vi "Read Compatible Hardware Table.vi"(8 "error in (no error)":errorcluster, 11 "Mag Lab Measure Controller in":refnum<class "Mag Lab Measure Controller.lvclass">) -> (0 "error out":errorcluster, 2 "Compatible Hardware Type Lookup Table (HardwareType -> DeviceNames[])":variant, 3 "Mag Lab Measure Controller out":refnum<class "Mag Lab Measure Controller.lvclass">)   [LabVIEW 2015, in "Mag Lab Measure Controller.lvclass"]
uses:
  Mag Lab Measure Controller.lvclass
  Mag Lab Measure Controller.lvclass/Mag Lab Measure Controller.ctl
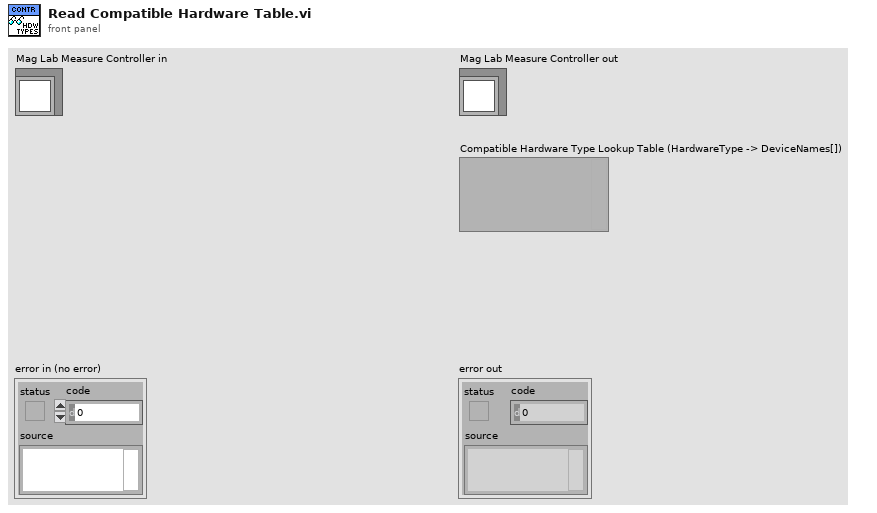
[diagram p1: front panel]
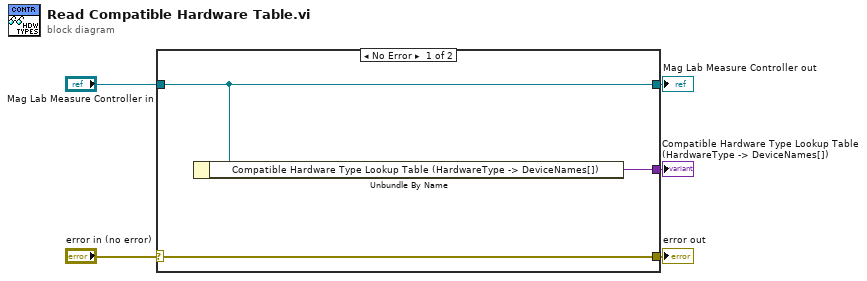
[diagram p0: block diagram]
diagram:
  n1 = case shown="No Error" "error in (no error)" {
    selector: "error in (no error)" -> [w8 w9]
    tunnel: [w8 w9] -> w4
    tunnel: [w7 w10] -> w2
    tunnel: "Mag Lab Measure Controller in" -> [w7 w10]
    tunnel: [w6 _] -> w1
    frame No Error {
      n2 = Unbundle By Name(w7) -> ("Compatible Hardware Type Lookup Table (HardwareType -> DeviceNames[])"=w6:variant)
    }
    frame Error {
    }
  }
  "error out" <- w4
  "Mag Lab Measure Controller out" <- w2
  "Compatible Hardware Type Lookup Table (HardwareType -> DeviceNames[])" <- w1
